vi "Aula2.vi"() -> ()   [LabVIEW 2020]
panel:
  in  "Numeric":dbl
  out "iterações 2":i32
  in  "ºF 2":dbl(slide) scale=0.0..110.0
  out "resultado\n 2":dbl
  out "ºC 2":dbl(slide) scale=0.0..100.0
  in  "stop 2":bool
  in  "Boolean":bool
  in  "stop":bool
  out "iterações":i32
  out "resultado":dbl
  out "ºC":dbl(slide) scale=0.0..100.0
  in  "ºF":dbl(slide) scale=0.0..110.0
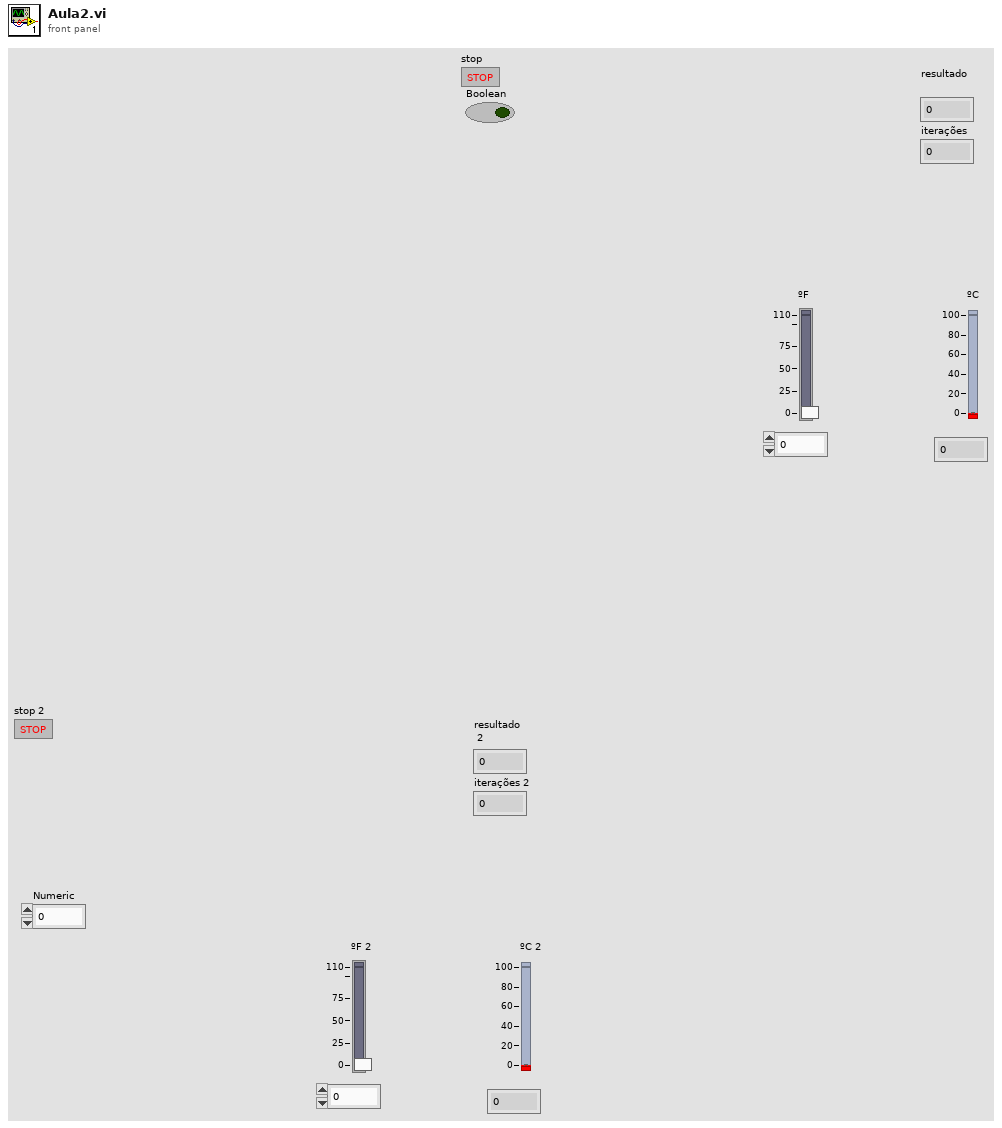
[diagram p1: front panel]
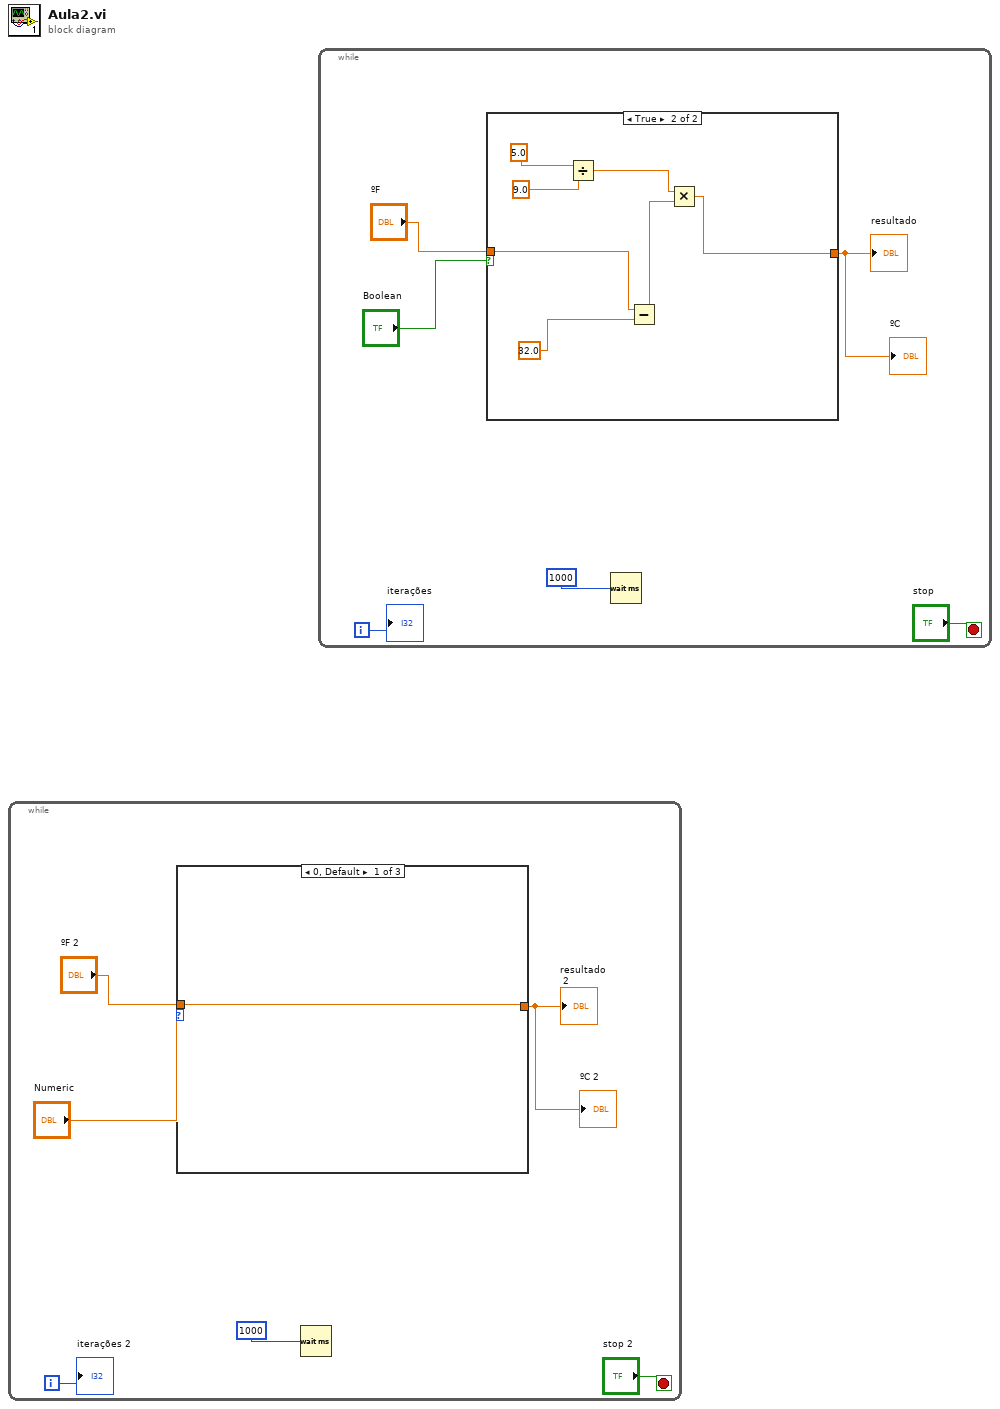
[diagram p0: block diagram]
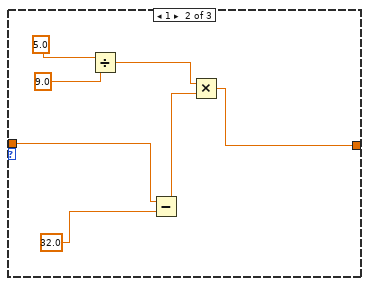
[diagram p2: hidden frame]
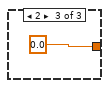
[diagram p3: hidden frame]
diagram:
  n1 = while {
    i -> [w5]
    stop <- "stop 2" stop-if-true
    n2 = case shown="0, Default" "Numeric" {
      tunnel: "ºF 2" -> [w7 w9 _]
      tunnel: [w7 w12 0.0 ("ºF 2")] -> w3
      frame 0, Default {
      }
      frame 1 {
        n3 = Divide(x=5.0, y=9.0) -> (x/y=w10:dbl)
        n4 = Subtract(x=w9, y=32.0 ("x")) -> (x-y=w11:dbl)
        n5 = Multiply(x=w10, y=w11) -> (x*y=w12:dbl)
      }
      frame 2 {
      }
    }
    "resultado\n 2" <- w3
    "ºC 2" <- w3
    n6 = Wait (ms)(milliseconds to wait=u32 1000 ("millisecond timer value")) -> ()  [unwired: 1 out]
    "iterações 2" <- w5
  }
  n7 = while {
    i -> [w20]
    stop <- "stop" stop-if-true
    n8 = case shown="True" "Boolean" {
      tunnel: "ºF" -> [w22 w24]
      tunnel: [w22 w27] -> w18
      frame False {
      }
      frame True {
        n9 = Divide(x=5.0, y=9.0) -> (x/y=w25:dbl)
        n10 = Subtract(x=w24, y=32.0 ("x")) -> (x-y=w26:dbl)
        n11 = Multiply(x=w25, y=w26) -> (x*y=w27:dbl)
      }
    }
    "resultado" <- w18
    "ºC" <- w18
    n12 = Wait (ms)(milliseconds to wait=u32 1000 ("millisecond timer value")) -> ()  [unwired: 1 out]
    "iterações" <- w20
  }
